vi "spatial_functional_global.vi"(4 "transformation description In":dbl[](array[numeric]), 5 "Update Translation Only":bool, 6 "Buffer Number":i32, 7 "Operation":T1) -> (0 "transformation description Out":dbl[](array[numeric]), 1 "all transformation descriptions Out":dbl[][](array[numeric]))   [LabVIEW 2019]
uses:
  SpatialFunctionalGlobalOperations.ctl
  ParametersGlobal.vi
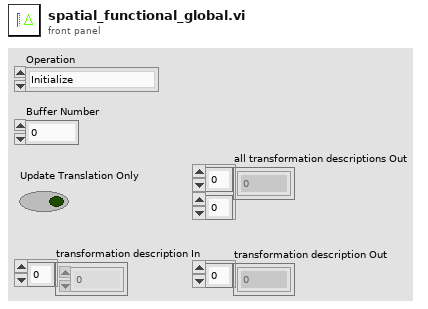
[diagram p1: front panel]
types:
  T1 = typedef "SpatialFunctionalGlobalOperations.ctl" = enum16{"Initialize", "Dump", "UpdateSpatialTransform", "ReadSpatialTransform"}
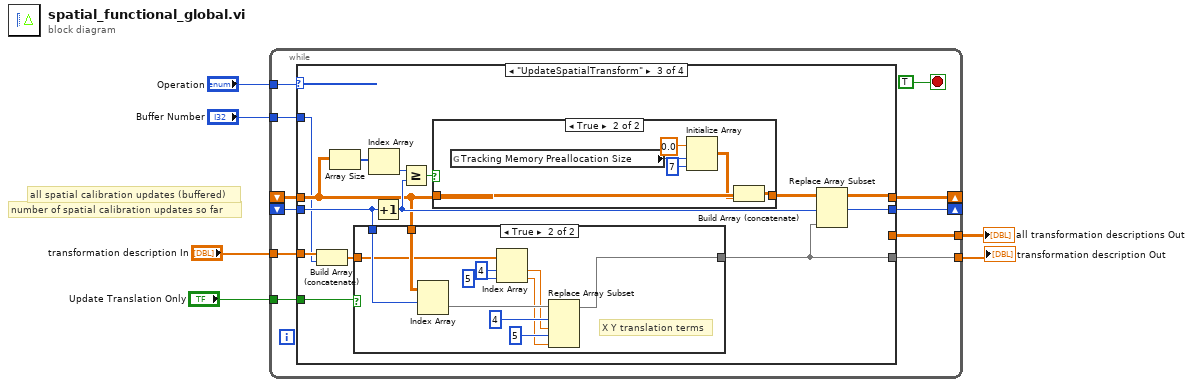
[diagram p0: block diagram]
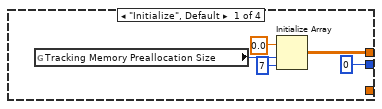
[diagram p2: hidden frame]
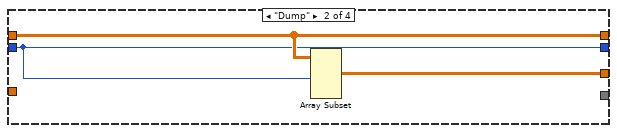
[diagram p3: hidden frame]
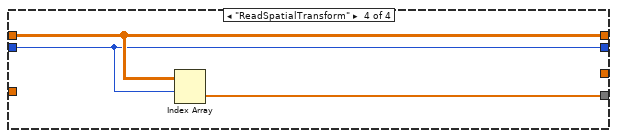
[diagram p6: hidden frame]
diagram:
  # "all spatial calibration updates (buffered)"
  # "number of spatial calibration updates so far"
  n1 = while {
    tunnel: "Operation" -> [w16]
    tunnel: "Buffer Number" -> [w15]
    tunnel: "transformation description In" -> [w12]
    shift-right: [w14] -> _
    shift-left: _ -> [w13]
    shift-right: [w11] -> _
    shift-left: _ -> [w10]
    tunnel: [w9] -> w3
    tunnel: [w8] -> w2
    tunnel: "Update Translation Only" -> [w7]
    stop <- TRUE stop-if-true
    n2 = case shown="\"UpdateSpatialTransform\"" w16 {
      tunnel: w15 -> [_ _ w27 _]
      tunnel: [w19 w25 w33 w59] -> w14
      tunnel: w13 -> [_ w25 w29 w59]
      tunnel: w12 -> [_ _ w28 _]
      tunnel: [0 ("Buffer Number Out") w23 w34 w58] -> w11
      tunnel: w10 -> [_ w23 w30 w58]
      tunnel: [_ w24 _ _] -> w9
      tunnel: [_ _ w32 w60] -> w8
      tunnel: w7 -> [_ _ w31 _]
      frame "Initialize", Default {
        n3 = global read "ParametersGlobal.vi" "Tracking Memory Preallocation Size"() -> (w22:i32)
        n4 = Initialize Array(0.0, w22, 7 ("dimension size")) -> (w19:dbl[][])
      }
      frame "Dump" {
        n5 = Array Subset(array=w25, length (row)=w23) -> (w24:dbl[][])  [unwired: 3 in]
      }
      frame "UpdateSpatialTransform" {
        n6 = Build Array (concatenate)(w28, w27) -> (w26:dbl[])
        n7 = Array Size(array=w29) -> (size(s)=w38:i32[])
        n8 = case shown="True" w31 {
          tunnel: [w39 w40] -> w32
          tunnel: w30 -> [_ w49]
          tunnel: w29 -> [_ w50]
          tunnel: w26 -> [w39 w45]
          frame False {
          }
          frame True {
            # "X Y translation terms"
            n9 = Index Array(array=w50, index (row)=w49) -> (element=w46:dbl[])  [unwired: 1 in]
            n10 = Index Array(array=w45, index #1=4 ("index"), index #2=5 ("index")) -> (element #1=w42:dbl, element #2=w41:dbl)
            n11 = Replace Array Subset(array=w46, new element #1=w42, index #1=4 ("index"), new element #2=w41, index #2=5 ("index")) -> (w40:dbl[])
          }
        }
        n12 = Index Array(array=w38) -> (element=w37:i32)  [unwired: 1 in]
        n13 = Increment(x=w30) -> (x+1=w34:i32)
        n14 = Greater Or Equal?(x=w37, y=w34) -> (x >= y?=w36:bool)
        n15 = case shown="True" w36 {
          tunnel: w29 -> [w51 w54]
          tunnel: [w51 w52] -> w35
          frame False {
          }
          frame True {
            n16 = global read "ParametersGlobal.vi" "Tracking Memory Preallocation Size"() -> (w57:i32)
            n17 = Initialize Array(0.0, w57, 7 ("dimension size")) -> (w53:dbl[][])
            n18 = Build Array (concatenate)(w54, w53) -> (w52:dbl[][])
          }
        }
        n19 = Replace Array Subset(array=w35, new element=w32, index (row)=w34) -> (w33:dbl[][])  [unwired: 1 in]
      }
      frame "ReadSpatialTransform" {
        n20 = Index Array(array=w59, index (row)=w58) -> (element=w60:dbl[])  [unwired: 1 in]
      }
    }
  }
  "all transformation descriptions Out" <- w3
  "transformation description Out" <- w2
